vi "SP Set Plot Channel Placement.vi"(3 "Split? (f = Overlay)":bool, 4 "ChIndex (0)":i32) -> (1 "Placement":T1)   [LabVIEW 2011]
uses:
  server/dd/lib/Report Templates/Template TDM/objPlacement.ctl
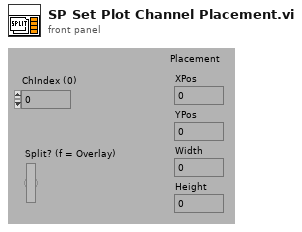
[diagram p1: front panel]
types:
  T1 = typedef "objPlacement.ctl" = cluster{"XPos":dbl, "YPos":dbl, "Width":dbl, "Height":dbl}
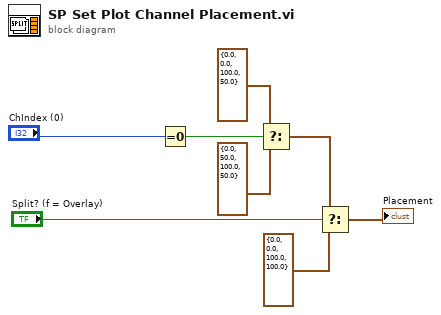
[diagram p0: block diagram]
diagram:
  n1 = Equal To 0?(x="ChIndex (0)") -> (x = 0?=w6:bool)
  n2 = Select(t=T1 {"XPos"=0.0, "YPos"=0.0, "Width"=100.0, "Height"=50.0} ("Placement"), s=w6, f=T1 {"XPos"=0.0, "YPos"=50.0, "Width"=100.0, "Height"=50.0} ("Placement")) -> (s? t:f=w2:T1)
  n3 = Select(t=w2, s="Split? (f = Overlay)", f=T1 {"XPos"=0.0, "YPos"=0.0, "Width"=100.0, "Height"=100.0} ("Placement")) -> (s? t:f=→"Placement":T1)
